vi "picoquant_open_device_handle.vi"(8 "error in (no error)":errorcluster, 11 "hydraharp in":refnum<class "hydraharp.lvclass">) -> (0 "error out":errorcluster, 3 "hydraharp out":refnum<class "hydraharp.lvclass">)   [LabVIEW 2015, in "hydraharp.lvclass"]
uses:
  hydraharp.lvclass
  hydraharp.lvclass/hydraharp.ctl
  hhlib.dll
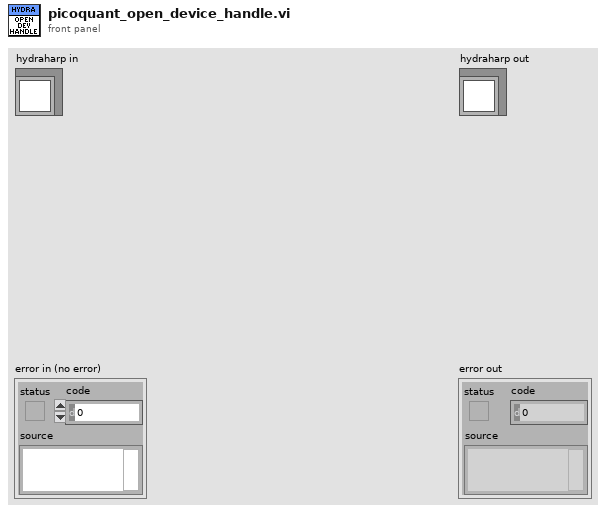
[diagram p1: front panel]
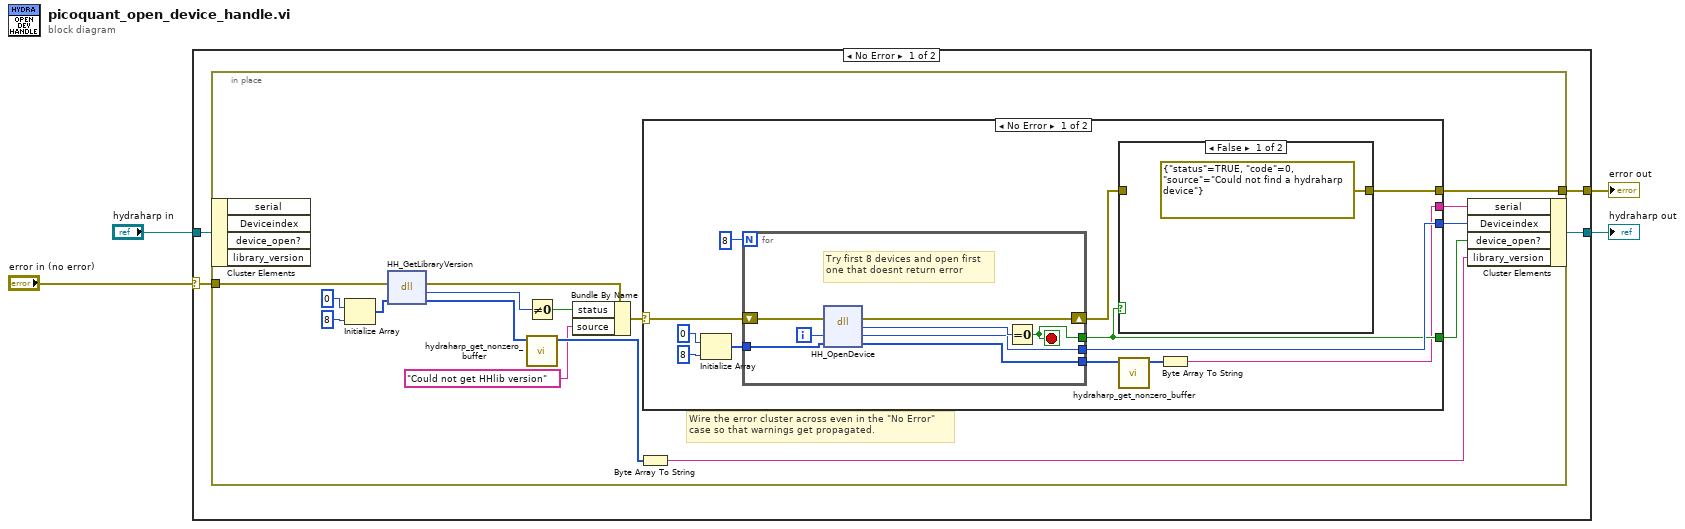
[diagram p0: block diagram]
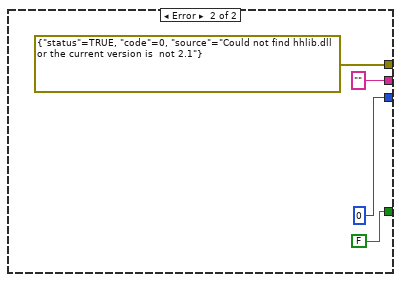
[diagram p3: hidden frame]
diagram:
  n1 = case shown="No Error" "error in (no error)" {
    selector: "error in (no error)" -> [w8 w52]
    tunnel: [w5 w52] -> w1
    tunnel: [w6 w51] -> w2
    tunnel: "hydraharp in" -> [w7 w51]
    frame No Error {
      n2 = in-place {
        in-place-border: w8 -> [w24]
        in-place-border: [w20] -> w5
        # "Wire the error cluster across even in the \"No Error\"\ncase so that warnings get propagated."
        n3 = in-place-cluster #1(w7) -> ()  [unwired: 4 out]
        n4 = Initialize Array(u8 0 ("element"), 8 ("dimension size")) -> (w17:u8[])
        n5 = dll-call lib="hhlib.dll" fn="HH_GetLibraryVersion"(error in=w24, "Version"=w17) -> (error out=w12:errorcluster, "return type"=w13:i32, "Version"=w16:u8[])  [unwired: 2 in, 1 out]
        n6 = Not Equal To 0?(x=w13) -> (x != 0?=w11:bool)
        n7 = call "hydraharp_get_nonzero_buffer.vi"("buffer"=w16) -> ("subarray"=w15:u8[])  [unwired: 10 in]
        n8 = Bundle By Name(cluster=w12, "status"=w11, "source"="Could not get HHlib version") -> (w9:errorcluster)
        n9 = Byte Array To String(unsigned byte array=w15) -> (string=w14:string)
        n10 = case shown="No Error" w9 {
          selector: w9 -> [w25 _]
          tunnel: [w27 "" ("serial")] -> w23
          tunnel: [w35 0 ("devidx")] -> w22
          tunnel: [w34 FALSE] -> w21
          tunnel: [w32 errorcluster {"status"=TRUE, "code"=0, "source"="Could not find hhlib.dll or the current version is  not 2.1"} ("error out")] -> w20
          frame No Error {
            n11 = Initialize Array(u8 0 ("element"), 8 ("dimension size")) -> (w29:u8[])
            n12 = for {
              N: 8 -> [_]
              tunnel: [w44] -> w26
              tunnel: [w42] -> w35
              tunnel: [w41] -> w34
              shift-right: [w40] -> w33
              shift-left: w25 -> [w46]
              tunnel: w29 -> [w39]
              i -> [w45]
              stop <- w41 stop-if-true
              # "Try first 8 devices and open first\none that doesnt return error"
              n13 = dll-call lib="hhlib.dll" fn="HH_OpenDevice"(error in=w46, "devidx"=w45, "serial"=w39) -> (error out=w40:errorcluster, "return type"=w43:i32, "devidx"=w42:i32, "serial"=w44:u8[])  [unwired: 2 in, 1 out]
              n14 = Equal To 0?(x=w43) -> (x = 0?=w41:bool)
            }
            n15 = case shown="False" w34 {
              tunnel: w33 -> [_ w38]
              tunnel: [errorcluster {"status"=TRUE, "code"=0, "source"="Could not find a hydraharp device"} ("error out") w38] -> w32
              frame False {
              }
              frame True {
              }
            }
            n16 = call "hydraharp_get_nonzero_buffer.vi"("buffer"=w26) -> ("subarray"=w28:u8[])  [unwired: 10 in]
            n17 = Byte Array To String(unsigned byte array=w28) -> (string=w27:string)
          }
          frame Error {
          }
        }
        n18 = in-place-cluster #1("serial"=w23, "Deviceindex"=w22, "device_open?"=w21, "library_version"=w14) -> (w6:refnum<class "hydraharp.lvclass">)
      }
    }
    frame Error {
    }
  }
  "error out" <- w1
  "hydraharp out" <- w2
